vi "lowest_col.vi"() -> ()   [LabVIEW 2017]
panel:
  out "Numeric":dbl
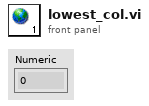
[diagram p1: front panel]
diagram:
